vi "PH_PILS.vis LaserEnablingKnob.vi"(0 "i ref in":refnum<vi>, 5 "error IO":errorcluster) -> (14 "i ref out":refnum<vi>, 19 "error out":errorcluster)   [LabVIEW 2014, in "PH_PILS.lvlib"]
uses:
  PH_PILS.lvlib
  PH_SystemInformation/PH_SystemInformation.lvlib
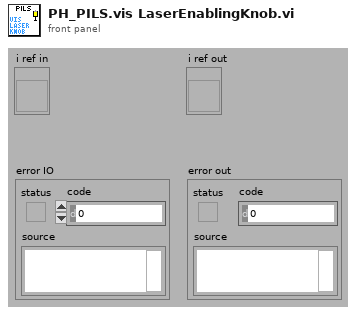
[diagram p1: front panel]
types:
  T1 = typedef "PH_PILS.lvlib/PH_PILS.i attribute.ctl" = cluster{"Boolean":cluster{"GUI Ref":refnum<vi>, "Status":i32}[], "GUI Refs Exp. Shutters":cluster{"1":refnum<vi>, "2":refnum<vi>, "3":refnum<vi>, "4":refnum<vi>}, "Tristate2Run GUI Refs":refnum<vi>[], "EO-Likes":cluster{"GUI Ref":refnum<vi>, "Status":i32}[], "Operation Mode":cluster{"Operation Mode":T2, "GUI":cluster{"Ref State":refnum<vi>, "Ref":refnum<vi>}, "Servicemode":cluster{"Tagname":string, "Status":i32}, "Labormode":cluster{"Tagname":string, "Status":i32}, "Searchmode":cluster{"Tagname":string, "Status":i32}, "Shotmode":cluster{"Tagname":string, "Status":i32}}, "Submode":cluster{"Submode":T3, "GUI":cluster{"Ref State":refnum<vi>, "Ref":refnum<vi>}, "Submode":cluster{"Tagname":string, "Status":i32}}, "Experiment":cluster{"Experiment":enum16{"unknown", "intern", "4 (Z6)", "3", "2", "1"}, "GUI":cluster{"Ref State":refnum<vi>, "Ref":refnum<vi>}, "intern":cluster{"Tagname":string, "Status":i32}, "Exp 4":cluster{"Tagname":string, "Status":i32}, "Exp 3":cluster{"Tagname":string, "Status":i32}, "Exp 2":cluster{"Tagname":string, "Status":i32}, "Exp 1":cluster{"Tagname":string, "Status":i32}}, "TristateNormal":cluster{"GUI Ref":refnum<vi>, "Status":i32}[], "Door Tags":cluster{"GUI Ref":refnum<vi>, "Status":i32}[], "GUIlessTags":cluster{"Name":string, "Status":i32}[], "Beamline GUI Refs":refnum<vi>[], "Special Boolean":cluster{"GUI Ref":refnum<vi>, "Status":i32}[], "Laserpower":cluster{"GUI Ref":refnum<vi>, "Status":i32}[], "Shutter":cluster{"GUI Ref":refnum<vi>, "Status":i32}[], "Tristate EO Like":cluster{"GUI Ref":refnum<vi>, "Status":i32}[], "PP":cluster{"GUI Ref":refnum<vi>, "Status":i32, "Head Ref":refnum<vi>, "Slider Ref":refnum<vi>}[], "Switch Knobs":cluster{"GUI Ref":refnum<vi>, "Status":i32}[], "Latch Knob GUI Refs":refnum<vi>[], "FailureCounter":i32, "Enabled Status":cluster{"Laser":i32, "PreAmp":i32, "MainAmp":i32}, "Mercury":refnum<vi>, "Instance Rods":string, "Logfile":path, "Beckhoff-Instance Internal":string, "Beckhoff-Instance External":string, "Enabling Rights":cluster{"Name":string, "Password":string, "PA?":bool, "MA?":bool, "Exp?":bool}[]}
  T2 = typedef "PH_PILS.lvlib/PH_PILS.Operation Mode.ctl" = enum16{"unknown", "Service", "Labor", "Search", "Shot"}
  T3 = typedef "PH_PILS.lvlib/PH_PILS.Submode.ctl" = enum16{"unknown", "HV-Normal", "HV-Test"}
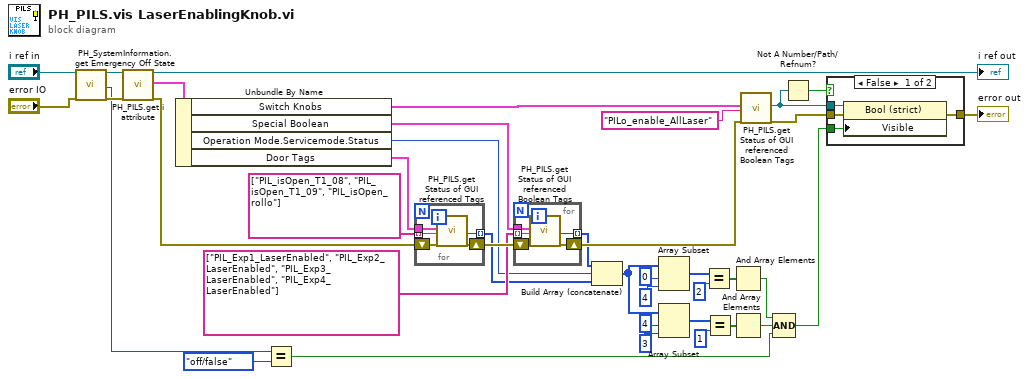
[diagram p0: block diagram]
diagram:
  n1 = call "PH_SystemInformation.get Emergency Off State.vi"("i ref in"="i ref in", "error in (no error)"="error IO") -> ("i ref out"=w4:refnum<vi>, "Emergency Off State"=w3:enum16{"no info", "off/false", "Alarm"}, "error out"=w6:errorcluster)  [unwired: 15 in]
  n2 = call "PH_PILS.get i attribute.vi"("i ref in"=w4, "error in (no error)"=w6) -> ("i ref out"=→"i ref out":refnum<vi>, "i attribute"=w29:T1, "error out"=w25:errorcluster)  [unwired: 15 in]
  n3 = Unbundle By Name(w29) -> ("Switch Knobs"=w28:cluster{"GUI Ref":refnum<vi>, "Status":i32}[], "Special Boolean"=w26:cluster{"GUI Ref":refnum<vi>, "Status":i32}[], "Operation Mode.Servicemode.Status"=w9:i32, "Door Tags"=w8:cluster{"GUI Ref":refnum<vi>, "Status":i32}[])
  n4 = Equal?(x=w3, y=enum16{"no info", "off/false", "Alarm"}."off/false") -> (x = y?=w1:bool)
  n5 = for {
    tunnel: string[] ["PIL_isOpen_T1_08", "PIL_isOpen_T1_09", "PIL_isOpen_rollo"] -> [w43] mode=indexing
    tunnel: [w44] -> w10 mode=indexing
    shift-right: [w42] -> w37
    shift-left: w25 -> [w41]
    tunnel: w8 -> [w40]
    n6 = call "PH_PILS.get Status of GUI referenced Tags.vi"("Tags"=w40, "Tagname"=w43, "error in"=w41) -> ("Status"=w44:i32, "error out"=w42:errorcluster)  [unwired: 13 in, 2 out]
  }
  n7 = for {
    tunnel: w26 -> [w47]
    tunnel: string[] ["PIL_Exp1_LaserEnabled", "PIL_Exp2_LaserEnabled", "PIL_Exp3_LaserEnabled", "PIL_Exp4_LaserEnabled"] -> [w46] mode=indexing
    shift-right: [w48] -> w24
    shift-left: w37 -> [w49]
    tunnel: [w45] -> w12 mode=indexing
    n8 = call "PH_PILS.get Status of GUI referenced Boolean Tags.vi"("Tags"=w47, "Tagname"=w46, "error in"=w49) -> ("Status"=w45:i32, "error out"=w48:errorcluster)  [unwired: 13 in, 2 out]
  }
  n9 = Build Array (concatenate)(w12, w9, w10) -> (w30:i32[])
  n10 = Array Subset(array=w30, index=0, length=4) -> (w33:i32[])
  n11 = Array Subset(array=w30, index=4, length=3) -> (w18:i32[])
  n12 = Equal?(x=w33, y=2) -> (x = y?=w17:bool[])
  n13 = Equal?(x=w18, y=1) -> (x = y?=w16:bool[])
  n14 = And Array Elements(Boolean array=w17) -> (logical AND=w15:bool)
  n15 = And Array Elements(Boolean array=w16) -> (logical AND=w14:bool)
  n16 = call "PH_PILS.get Status of GUI referenced Boolean Tags.vi"("Tags"=w28, "Tagname"="PILo_enable_AllLaser", "error in"=w24) -> ("GUI Ref"=w22:refnum<vi>, "error out"=w27:errorcluster)  [unwired: 13 in, 2 out]
  n17 = Compound Arithmetic op=AND(w15, w14, w1) -> (w13:bool)
  n18 = Not A Number/Path/Refnum?(number/path/refnum=w22) -> (NaN/Path/Refnum?=w23:bool)
  n19 = case shown="False" w23 {
    tunnel: w27 -> [w53 w54]
    tunnel: w22 -> [w52 _]
    tunnel: [w51 w54] -> w21
    tunnel: w13 -> [w50 _]
    frame False {
      n20 = property class="Bool (strict)"(reference=w52, error in=w53, "Visible"=w50) -> (error out=w51:errorcluster)  [unwired: 1 out]
    }
    frame True {
    }
  }
  "error out" <- w21
